vi "SwissSPAD Live_Get FPGA Data Q.vi"(1 "create if not found? (T)":bool, 4 "error in (no error)":errorcluster, 6 "FPGA Data Q Name":string) -> (5 "error out":errorcluster, 7 "FPGA Data Q":refnum<queue>)   [LabVIEW 2021]
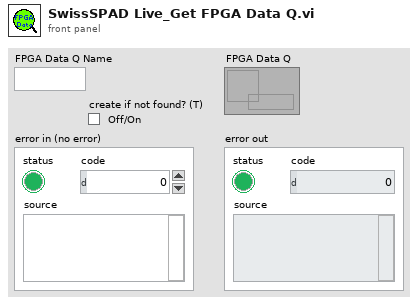
[diagram p1: front panel]
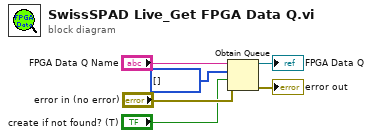
[diagram p0: block diagram]
diagram:
  n1 = Obtain Queue(name (unnamed)="FPGA Data Q Name", element data type=u8[] [] ("BYTEARRAY"), create if not found? (T)="create if not found? (T)", error in (no error)="error in (no error)") -> (queue out=→"FPGA Data Q":refnum<queue>, error out=→"error out":errorcluster)  [unwired: 1 in, 1 out]
